vi "Saving_LOG.vi"(0 "Path":path, 5 "Report":string, 7 "Report AURA":string, 9 "Path Carpeta":path, 11 "Nº Archivos Max":i32) -> (4 "path":path, 15 "Report":string)   [LabVIEW 2015]
panel:
  out "error out":errorcluster
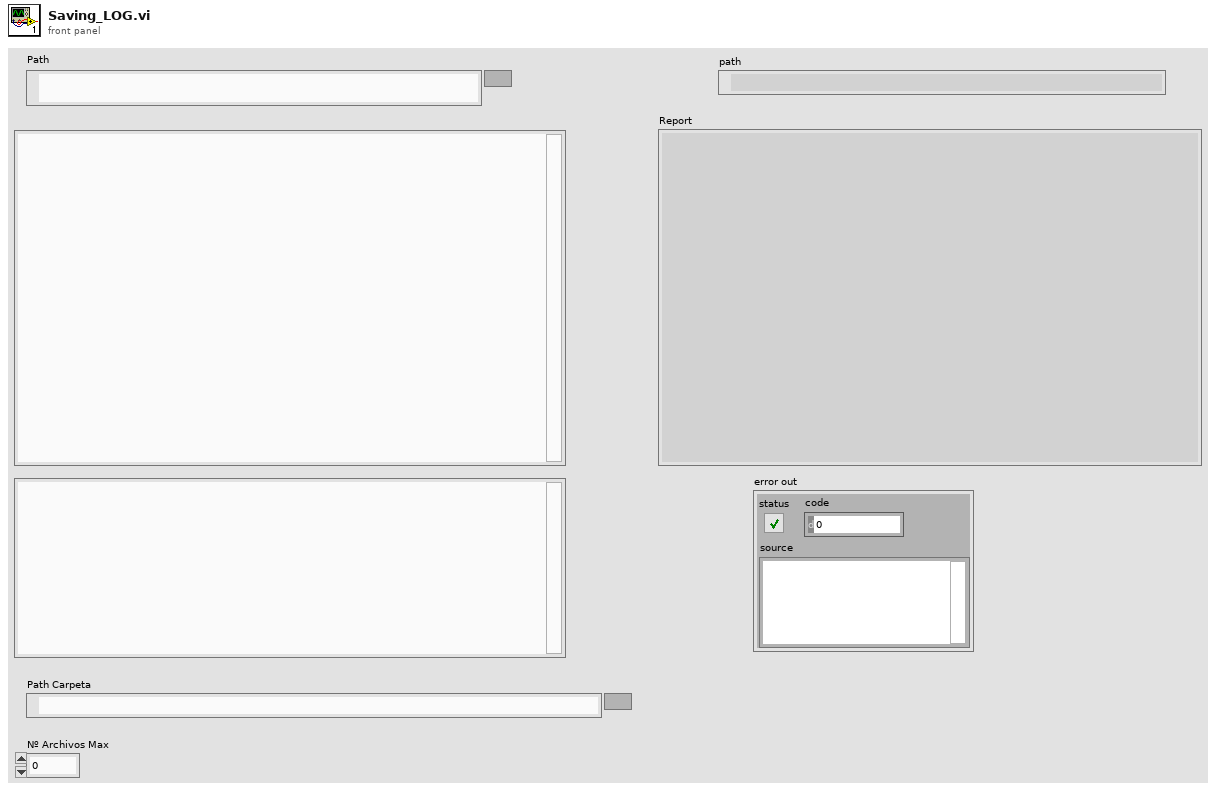
[diagram p1: front panel]
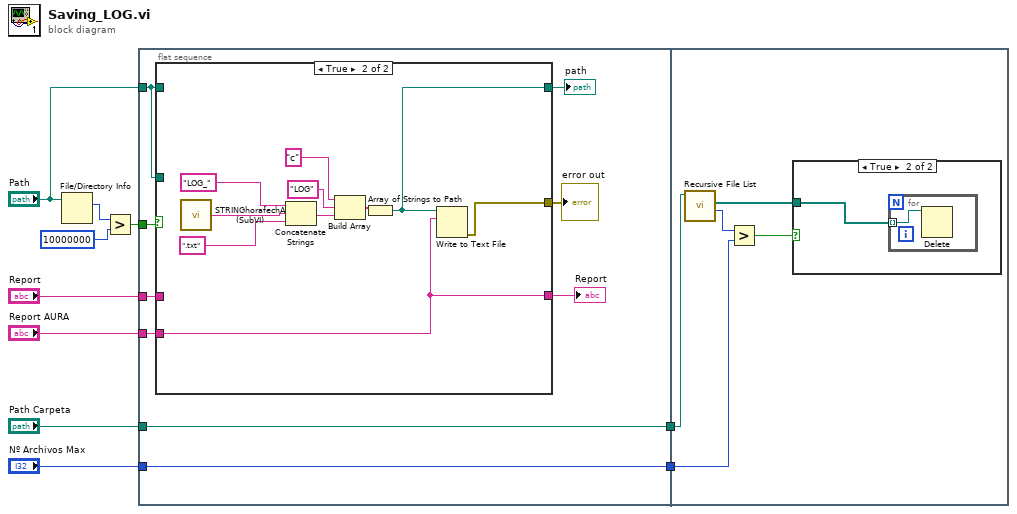
[diagram p0: block diagram]
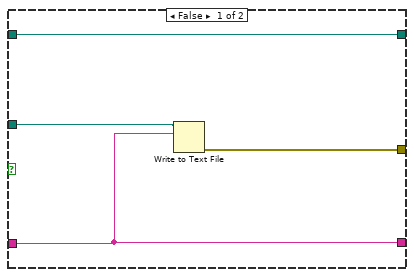
[diagram p2: hidden frame]
diagram:
  n1 = File/Directory Info(path="Path") -> (size=w10:i64)  [unwired: 1 in, 6 out]
  n2 = Greater?(x=w10, y=i64 10000000) -> (0:w8:bool)
  n3 = flat-sequence {
    tunnel: w8 -> [w19]
    tunnel: "Report AURA" -> [w18]
    tunnel: "Report" -> [w17]
    tunnel: "Path" -> [w16]
    tunnel: "Path Carpeta" -> [w12]
    tunnel: [w12] -> w3
    tunnel: "Nº Archivos Max" -> [w11]
    tunnel: [w11] -> w1
    tunnel: w3 -> [w35]
    tunnel: w1 -> [w34]
    frame #0 {
      n4 = case shown="True" w19 {
        tunnel: [w23 w27] -> w15
        tunnel: w18 -> [_ w26]
        tunnel: [w21 w26] -> w13
        tunnel: w16 -> [w23 _]
        tunnel: w17 -> [w21 _]
        tunnel: w16 -> [w22 _]
        tunnel: [w20 w25] -> w14
        frame False {
          n5 = Write to Text File(file (use dialog)=w22, text=w21) -> (error out=w20:errorcluster)  [unwired: 2 in, 2 out]
        }
        frame True {
          n6 = call "STRINGhorafechA(SubVI).vi"() -> ("STRINGhora_fecha"=w31:string)
          n7 = Concatenate Strings("LOG_" ("string"), w31, ".txt" ("string")) -> (w33:string)
          n8 = Build Array("c", "LOG" ("element"), w33) -> (w30:string[])
          n9 = Array of Strings to Path(0:w30) -> (2:w27:path)  [unwired: 1 out]
          n10 = Write to Text File(file (use dialog)=w27, text=w26) -> (error out=w25:errorcluster)  [unwired: 1 in, 3 out]
        }
      }
      "path" <- w15
      "error out" <- w14
      "Report" <- w13
    }
    frame #1 {
      n11 = call <vilib>:"Recursive File List.vi"("Folder Path"=w35) -> ("Number of Files"=w37:i32, "All Files in Dir"=w36:path[])  [unwired: 6 in, 3 out]
      n12 = Greater?(x=w37, y=w34) -> (0:w38:bool)
      n13 = case shown="True" w38 {
        tunnel: w36 -> [_ w39]
        frame False {
        }
        frame True {
          n14 = for {
            tunnel: w39 -> [w40] mode=indexing
            n15 = Delete(path (use dialog)=w40) -> ()  [unwired: 4 in, 3 out]
          }
        }
      }
    }
  }
